vi "PathPlanner_TrajectoryEvent_New_Cmd.vi"(10 "Command":T2, 11 "Time_Secs":dbl) -> (3 "TrajectoryEvent":T1)   [LabVIEW 2019, in "PathPlanner24.lvlib"]
uses:
  PathPlanner24.lvlib
  ENum/PathPlanner_CommandUtil_Type_ENUM.ctl
  TypeDef/PathPlannerCommandUtil.ctl
  TypeDef/PathPlannerTrajectoryEvent.ctl
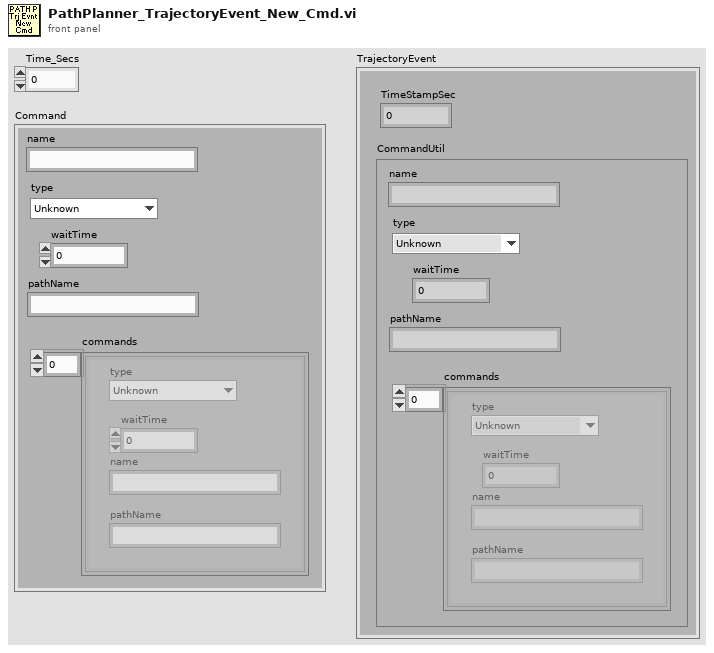
[diagram p1: front panel]
types:
  T1 = typedef "PathPlanner24.lvlib/PathPlannerTrajectoryEvent.ctl" = cluster{"TimeStampSec":dbl, "CommandUtil":T2}
  T2 = typedef "PathPlanner24.lvlib/PathPlannerCommandUtil.ctl" = cluster{"waitTime":dbl, "name":string, "pathName":string, "commands":cluster{"type":T3, "waitTime":dbl, "name":string, "pathName":string}[], "type":T3}
  T3 = typedef "PathPlanner24.lvlib/PathPlanner_CommandUtil_Type_ENUM.ctl" = enum16{"Unknown", "Wait", "Named", "Path", "Sequential", "Parallel", "Race", "Deadline", "PointTowardsZoneEnter", "PointTowardsZoneExit", "TriggerEventStart", "TriggerEventStop", "TriggerEventOneshot"}
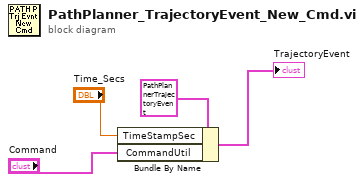
[diagram p0: block diagram]
diagram:
  n1 = Bundle By Name(cluster=T1 {"TimeStampSec"=0.0, "CommandUtil"={"waitTime"=0.0, "name"="", "pathName"="", "commands"=[], "type"=enum."Unknown"}} ("TrajectoryEvent"), "TimeStampSec"="Time_Secs", "CommandUtil"="Command") -> (→"TrajectoryEvent":T1)
